vi "Get Allocated Image Count.vi"() -> (0 "Number of allocated images":i16)   [LabVIEW 2011, in "labvvis.lvlib"]
doc: "Returns the number of images allocated. After your program terminates, this number should be zero. Any non-zero value indicates that an image was not deleted.\n\nIf an image was not deleted when it should have been, you will need to restart LabVIEW in order for this VI to return 0."
uses:
  <userlib>/labvvis/labvvis.lvlib
  labvvis.framework
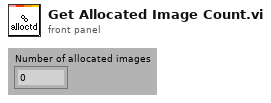
[diagram p1: front panel]
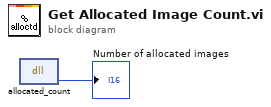
[diagram p0: block diagram]
diagram:
  n1 = dll-call lib="labvvis.framework" fn="allocated_count"() -> (→"Number of allocated images":i16)  [unwired: 3 in, 2 out]
